vi "PWM Scale.vi"(6 "Output Range":T1={"output low"=-8.0, "output high"=8.0} caption="output range", 7 "Max. Duty Cycle (0-2000)":fxp<+/-,16,16>=2000.0, 11 "Current Setpoint":fxp<+/-,18,6> format="%#_14g") -> (3 "Scaled Duty Cycle (0-2000)":i16)   [LabVIEW 2015]
uses:
  <vilib>/Motion/MotorControl/_s/nism.pi.v.outputRange.fxp.6.12.ctl
  <vilib>/Platform/TimedLoop/XDataNode/timing_clust.ctl
  <vilib>/Platform/TimedLoop/XDataNode/nitl_modes.ctl
  <vilib>/Platform/TimedLoop/XDataNode/wakeup.ctl
  <vilib>/rvi/FXPMathLib/FxpDiv/subVIs/nifxpmath_Div_SimConfig.ctl
  <vilib>/rvi/FXPMathLib/FxpDiv/simVIs/DllFxpDivTemp_sub.vi
  <vilib>/rvi/Emulation/niFpgaSctlEmulationGetInTimedLoop.vi
  <vilib>/rvi/Emulation/niFpgaEmulationReportErrorSimple.vi
  <vilib>/rvi/Emulation/niFpgaGetClockAttributes.vi
  <vilib>/rvi/Emulation/niFpgaCriticalErrorInLSC.vi
  <vilib>/rvi/FXPMathLib/FxpDiv/XNode/nifxpmath_Div.xnode
  <vilib>/rvi/FXPMathLib/FxpMul/XNode/nifxpmath_Multiplier.xnode
  <vilib>/Platform/TimedLoop/XDataNode/XDataNode.xnode
  <vilib>/rvi/FXPMathLib/sim/FxpSim.dll
  <vilib>/Platform/TimedLoop/XDataNode/XDNodeRunTimeDep.lvlib
  <vilib>/Motion/MotorControl/NI_SoftMotion_MotorControlIP.lvlib
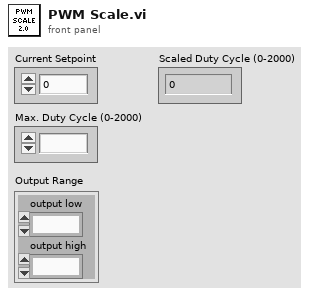
[diagram p1: front panel]
types:
  T1 = typedef "NI_SoftMotion_MotorControlIP.lvlib/nism.pi.v.outputRange.fxp.6.12.ctl" = cluster{"output low":fxp<+/-,18,6>, "output high":fxp<+/-,18,6>}
  T2 = typedef "XDNodeRunTimeDep.lvlib/timing_clust.ctl" = cluster{"Expected End [f-1]":u64, "Actual End [f-1]":u64, "Finished Late? [f-1]":bool, "Expected End [i-1]":u64, "Actual End [i-1]":u64, "Finished Late? [i-1]":bool, "Expected Start [i]":u64, "Actual Start [i]":u64, "Expected Start [f]":u64, "Actual Start [f]":u64, "Source Name":string, "Structure Name":string, "Period":i64, "Deadline":i64, "Offset":i64, "Start":i64, "Priority":i32, "Timeout":i32, "Mode":T3, "Wakeup Reason":T4, "Error":errorcluster, "Source Type":string, "Secondary Source Type":string, "Global End Time":u64, "Global Start Time":u64, "Frame Duration":u64, "Iteration Duration":u64, "Assigned CPU":i32, "I/O Scan Engine Mode":u32}
  T3 = typedef "XDNodeRunTimeDep.lvlib/nitl_modes.ctl" = enum32{"No Change", "Process missed periods, maintain original phase", "Discard missed periods, maintain original phase", "Process missed periods, ignore original phase", "Discard missed periods, ignore original phase"}
  T4 = typedef "XDNodeRunTimeDep.lvlib/wakeup.ctl" = enum32{"Normal", "Aborted", "Asynchronous wakeup", "Timing source error", "Timed loop error", "Timeout"}
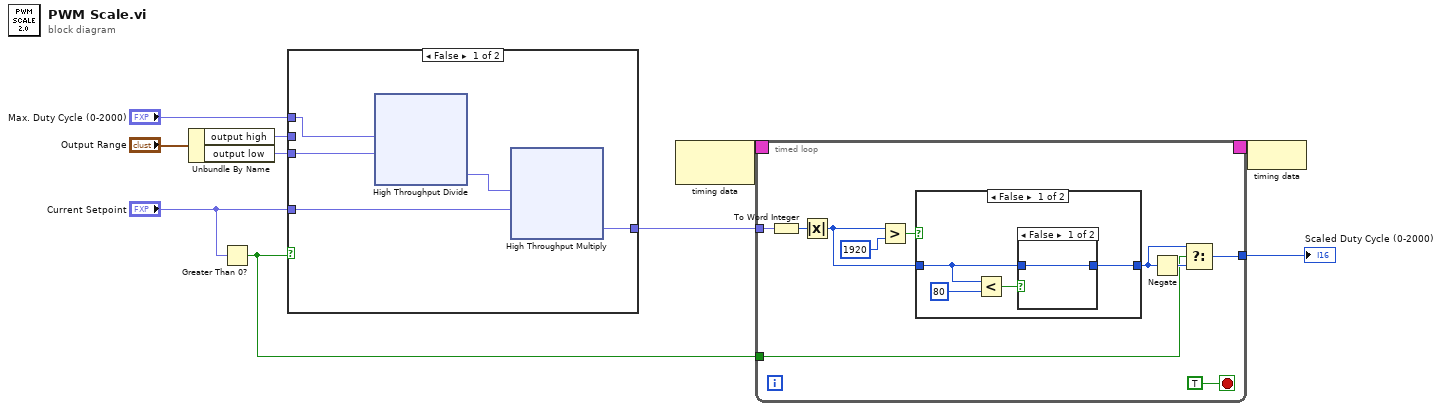
[diagram p0: block diagram]
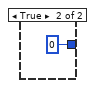
[diagram p2: hidden frame]
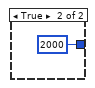
[diagram p3: hidden frame]
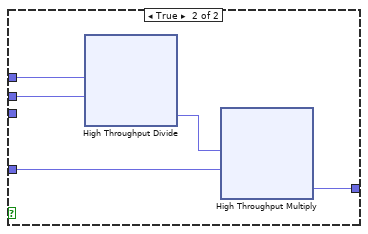
[diagram p4: hidden frame]
diagram:
  n1 = Unbundle By Name("Output Range") -> ("output high"=w8:fxp<+/-,18,6>, "output low"=w7:fxp<+/-,18,6>)
  n2 = Greater Than 0?(x="Current Setpoint") -> (x > 0?=w3:bool)
  n3 = case shown="False" w3 {
    tunnel: w8 -> [_ w45]
    tunnel: w7 -> [w13 _]
    tunnel: "Max. Duty Cycle (0-2000)" -> [w14 w46]
    tunnel: "Current Setpoint" -> [w12 w44]
    tunnel: [w11 w43] -> w4
    frame False {
      n4 = xnode "High Throughput Divide"("x"=w14, "y"=w13) -> ("x/y"=w15:fxp<+/-,28,28>)
      n5 = xnode "High Throughput Multiply"("x"=w15, "y"=w12) -> ("x*y"=w11:fxp<+/-,46,34>)
    }
    frame True {
      n6 = xnode "High Throughput Divide"("x"=w46, "y"=w45) -> ("x/y"=w47:fxp<+/-,28,28>)
      n7 = xnode "High Throughput Multiply"("x"=w47, "y"=w44) -> ("x*y"=w43:fxp<+/-,46,34>)
    }
  }
  n8 = node-c288() -> (w2:T2)  [unwired: 1 in]
  n9 = timed-loop {
    timing: w2 -> [_]
    timing-out: [_] -> w1
    tunnel: [w84] -> w10
    tunnel: w4 -> [w78]
    tunnel: w3 -> [w76]
    stop <- TRUE stop-if-true
    n10 = To Word Integer(number=w78) -> (16bit integer=w77:i16)
    n11 = Absolute Value(x=w77) -> (abs(x)=w81:i16)
    n12 = Greater?(x=w81, y=i16 1920) -> (0:w82:bool)
    n13 = case shown="False" w82 {
      tunnel: w81 -> [w86 _]
      tunnel: [w85 i16 2000] -> w79
      frame False {
        n14 = Less?(x=w86, y=i16 80) -> (x < y?=w87:bool)
        n15 = case shown="False" w87 {
          tunnel: w86 -> [w89 _]
          tunnel: [w89 i16 0] -> w85
          frame False {
          }
          frame True {
          }
        }
      }
      frame True {
      }
    }
    n16 = Negate(x=w79) -> (-x=w80:i16)
    n17 = Select(t=w79, s=w76, f=w80) -> (s? t:f=w84:i16)
  }
  "Scaled Duty Cycle (0-2000)" <- w10
  n18 = node-c288(w1) -> ()
